vi "Apply.vi"(8 "error in (no error)":errorcluster, 9 "Vmax":dbl, 10 "Array in":dbl[](array[numeric]), 11 "Level in":refnum<class "Level.lvclass">) -> (0 "error out":errorcluster, 2 "Array out":dbl[](array[numeric]), 3 "Level out":refnum<class "Level.lvclass">)   [LabVIEW 2020, in "Level.lvclass"]
uses:
  Level.lvclass
  Level.lvclass/Level.ctl
  3af96ae1-0caf-414a-9161-2a80d9c15747.vi
  98da9008-ef56-4d64-91a3-47755f63d727.vi
panel:
  in  "Apply multiplier? (F)":bool
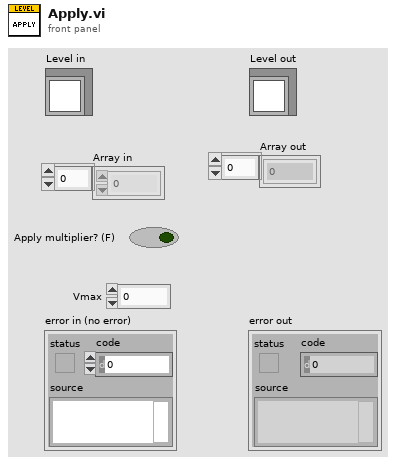
[diagram p1: front panel]
types:
  T1 = typedef "Level.lvclass/LevelUnits.ctl" = enum16{"dB atten", "dB SPL", "dB Vrms", "Volts", "dB mW", "mW", "dB HL", "dB SL"}
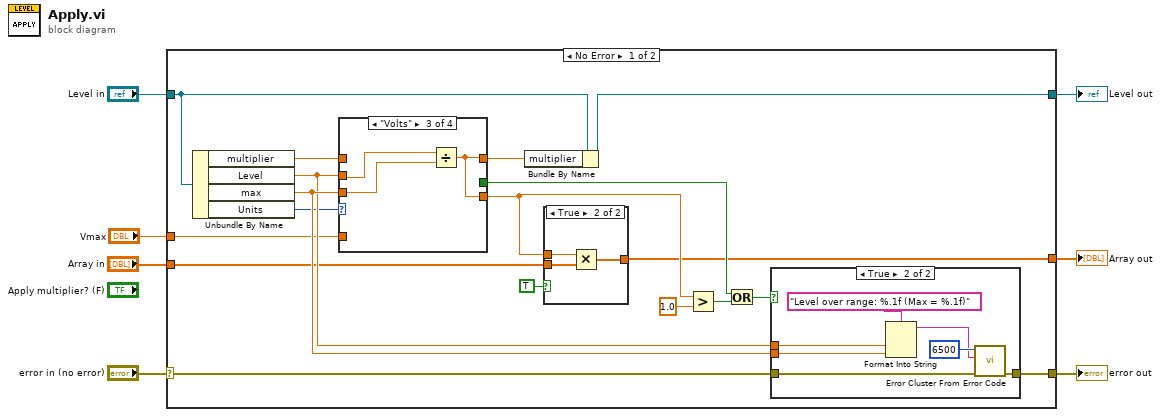
[diagram p0: block diagram]
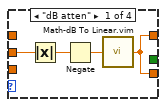
[diagram p4: hidden frame]
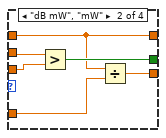
[diagram p5: hidden frame]
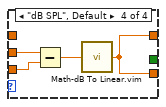
[diagram p6: hidden frame]
diagram:
  n1 = case shown="No Error" "error in (no error)" {
    selector: "error in (no error)" -> [w11 w55]
    tunnel: [w12 w55] -> w6
    tunnel: [w15 w54] -> w4
    tunnel: "Level in" -> [w16 w54]
    tunnel: "Array in" -> [w14 _]
    tunnel: [w13 _] -> w2
    tunnel: "Vmax" -> [w9 _]
    frame No Error {
      n2 = Unbundle By Name(w16) -> ("multiplier"=w23:dbl, "Level"=w20:dbl, "max"=w21:dbl, "Units"=w17:T1)
      n3 = case shown="\"Volts\"" w17 {
        tunnel: w21 -> [_ w45 w47 w53]
        tunnel: w20 -> [w40 w46 w49 w51]
        tunnel: [w37 w43 w48 w50] -> w22
        tunnel: w23 -> [_ w41 _ _]
        tunnel: [_ w44 _ _] -> w25
        tunnel: w9 -> [_ w42 _ _]
        tunnel: [w37 w41 w48 w50] -> w8
        frame "dB atten" {
          n4 = Absolute Value(x=w40) -> (abs(x)=w39:dbl)
          n5 = Negate(x=w39) -> (-x=w38:dbl)
          n6 = call "Math-dB To Linear.vim"("dB"=w38) -> ("linear"=w37:dbl)
        }
        frame "dB mW", "mW" {
          n7 = Greater?(x=w46, y=w45) -> (0:w44:bool)
          n8 = Divide(x=w41, y=w42) -> (x/y=w43:dbl)
        }
        frame "Volts" {
          n9 = Divide(x=w49, y=w47) -> (x/y=w48:dbl)
        }
        frame "dB SPL", Default {
          n10 = Subtract(x=w51, y=w53) -> (x-y=w52:dbl)
          n11 = call "Math-dB To Linear.vim"("dB"=w52) -> ("linear"=w50:dbl)
        }
      }
      n12 = Bundle By Name(cluster=w16, "multiplier"=w8) -> (w15:refnum<class "Level.lvclass">)
      n13 = case shown="True" TRUE {
        tunnel: w14 -> [w33 w36]
        tunnel: w22 -> [_ w35]
        tunnel: [w33 w34] -> w13
        frame False {
        }
        frame True {
          n14 = Multiply(x=w35, y=w36) -> (x*y=w34:dbl[])
        }
      }
      n15 = Greater?(x=w22, y=1.0) -> (0:w19:bool)
      n16 = Or(x=w25, y=w19) -> (x .or. y?=w24:bool)
      n17 = case shown="True" w24 {
        tunnel: [_ w32] -> w12
        tunnel: w20 -> [_ w27]
        tunnel: w21 -> [_ w29]
        tunnel: w11 -> [_ w26]
        frame False {
        }
        frame True {
          n18 = Format Into String(format string="Level over range: %.1f (Max = %.1f)", w27, w29) -> (resulting string=w28:string)  [unwired: 2 in, 1 out]
          n19 = call <vilib>:"Error Cluster From Error Code.vi"("error in (no error)"=w26, "error message (\"\")"=w28, "error code (0)"=6500) -> ("error out"=w32:errorcluster)  [unwired: 6 in]
        }
      }
    }
    frame Error {
    }
  }
  "error out" <- w6
  "Level out" <- w4
  "Array out" <- w2
